vi "Multipoint SMU Read.vi"() -> ()   [LabVIEW 2010]
uses:
  <instrlib>/Keithley 2400/Keithley 24XX.lvlib
panel:
  out "Waveform Chart":sgl[](graph)
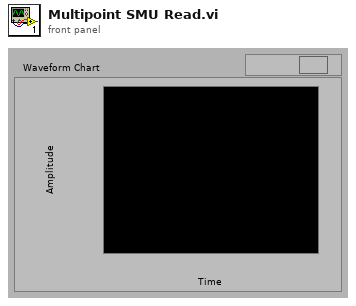
[diagram p1: front panel]
types:
  T1 = enum16{"--Disconnect All--", "Connect PulseGen to CH1", "Connect PulseGen to CH2", "Connect PulseGen to CH3", "Connect PulseGen to CH4", "Connect PulseGen to CH5", "Connect PulseGen to CH6", "Connect PulseGen to CH7", "Connect PulseGen to CH8", "Connect PulseGen to CH9", "Connect PulseGen to CH10", "Connect PulseGen to CH11", "Connect PulseGen to CH12", "Connect PulseGen to CH13", "Connect PulseGen to CH14", "Connect PulseGen to CH15", "Connect PulseGen to CH16", "Connect PulseGen to CH17", "Connect PulseGen to CH18", "Connect PulseGen to CH19", "Connect PulseGen to CH20", "Connect PulseGen to CH21", "Connect PulseGen to CH22", "Connect PulseGen to CH23", "Connect PulseGen to CH24", "Connect PulseGen to CH25", "Set MAG_SW", "Set Dynamic Load", "Set Expansion Trigger", "Trigger Positive Pulse", "Trigger Negative Pulse", "Set MSP Magic Pin", "Set BAT_EN", "Connect MSP_ACLK to CTR", "Connect MSP_MCLK to CTR", "Connect MSP_DIG_TST_OUT to CTR", "Connect STIM_SCK to CTR", "Connect STIM_CLK to CTR", "Connect SMU2 to Magnet", "Magnet Enable", "Cap Short", "Connect Positive Pulse to Pulse Bus", "Connect Negative Pulse to Pulse Bus", "Connect JTAG", "Connect JTAG DVDD Power", "RF Attach", "Connect SMU3 to VBAT", "Connect SMU3 Soft Start", "Connect ARB to Charge Coil", "Connect ARB to Matrix", "Connect CTR to Matrix", "DMM_I Short", "DMM_I 1000 Ohm", "DMM_I 100 Ohm", "DMM_I 10 Ohm", "Connect CH25 to DUT GND"}
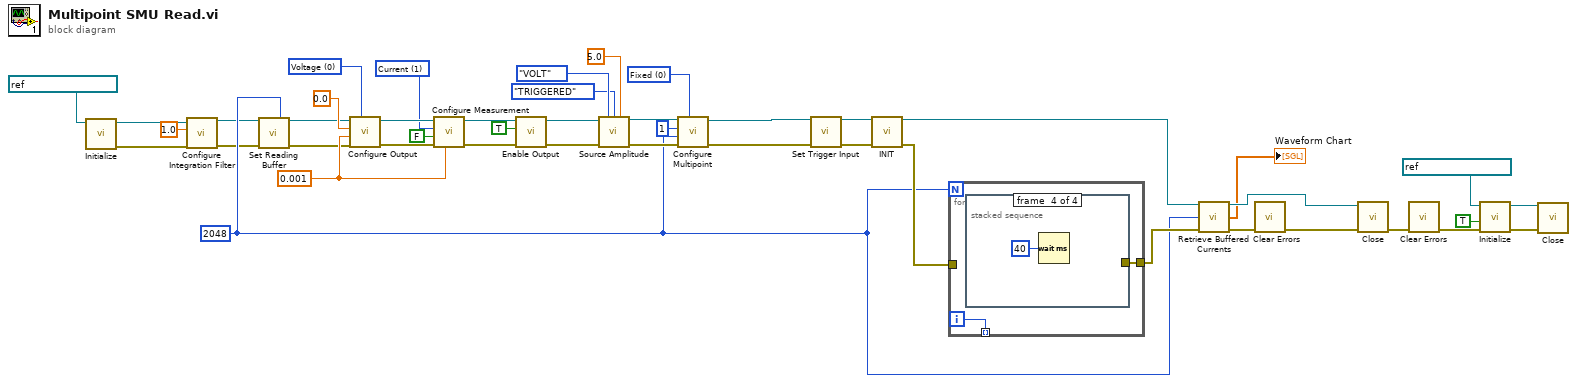
[diagram p0: block diagram]
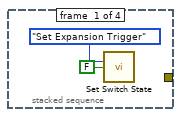
[diagram p2: hidden frame]
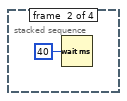
[diagram p3: hidden frame]
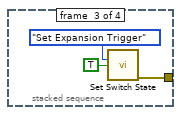
[diagram p4: hidden frame]
diagram:
  w3 = 2048 ("Reading Count")
  w26 = u16 0 items=["Fixed", "Sweep", "List"] ("Output Mode (0: Fixed)")
  w33 = u16 1 items=["Volts", "Current", "Resistance"] ("Function (0: Volts)")
  w34 = u16 0 items=["Voltage", "Current"] ("Source Mode  (0: Voltage)")
  w31 = 0.001 ("Compliance  Level (0.1)")
  n1 = call <instrlib>:"Initialize.vi"("VISA resource name"=refnum<visa-resource-name> "GPIB0::9::INSTR") -> ("error out"=w43:errorcluster, "VISA resource name out"=w45:refnum<visa-resource-name>)  [unwired: 9 in]
  n2 = call <instrlib>:"Configure Integration Filter.vi"("error in (no error)"=w43, "Measurement Speed (1 PLC)"=1.0, "VISA resource name"=w45) -> ("error out"=w1:errorcluster, "VISA resource name out"=w2:refnum<visa-resource-name>)  [unwired: 7 in]
  n3 = call "Set Reading Buffer.vi"("VISA resource name"=w2, "Reading Count"=w3, "error in (no error)"=w1) -> ("VISA resource name out"=w8:refnum<visa-resource-name>, "error out"=w7:errorcluster)  [unwired: 11 in]
  n4 = call <instrlib>:"Configure Output.vi"("Source Mode  (0: Voltage)"=w34, "error in (no error)"=w7, "Compliance  Level (0.1)"=w31, "Output Level (0)"=0.0, "VISA resource name"=w8) -> ("error out"=w41:errorcluster, "VISA resource name out"=w38:refnum<visa-resource-name>)  [unwired: 5 in]
  n5 = call <instrlib>:"Configure Measurement.vi"("Manual Range (1.0)"=w31, "error in (no error)"=w41, "Enable Auto Range (T:Enable)"=FALSE, "Function (0: Volts)"=w33, "VISA resource name"=w38) -> ("error out"=w40:errorcluster, "VISA resource name out"=w37:refnum<visa-resource-name>)  [unwired: 5 in]
  n6 = call <instrlib>:"Enable Output.vi"("error in (no error)"=w40, "Enable Output (T: Enable)"=TRUE, "VISA resource name"=w37) -> ("error out"=w39:errorcluster, "VISA resource name out"=w36:refnum<visa-resource-name>)  [unwired: 7 in]
  n7 = call "Source Amplitude.vi"("VISA resource name"=w36, "Source Function"=enum16{"CURR", "VOLT"}."VOLT", "Mode"=enum16{"IMM", "TRIGGERED"}."TRIGGERED", "Source Level"=5.0, "error in (no error)"=w39) -> ("VISA resource name out"=w25:refnum<visa-resource-name>, "error out"=w24:errorcluster)  [unwired: 9 in]
  n8 = call <instrlib>:"Configure Multipoint.vi"("Output Mode (0: Fixed)"=w26, "error in (no error)"=w24, "Trigger Count (1)"=w3, "Number of Times to Arm (1)"=1, "VISA resource name"=w25) -> ("error out"=w5:errorcluster, "VISA resource name out"=w6:refnum<visa-resource-name>)  [unwired: 5 in]
  n9 = call "Set Trigger Input.vi"("VISA resource name"=w6, "error in (no error)"=w5) -> ("VISA resource name out"=w21:refnum<visa-resource-name>, "error out"=w20:errorcluster)  [unwired: 12 in]
  n10 = call "INIT.vi"("VISA resource name"=w21, "error in (no error)"=w20) -> ("VISA resource name out"=w9:refnum<visa-resource-name>, "error out"=w23:errorcluster)  [unwired: 12 in]
  n11 = for {
    N: w3 -> [_]
    tunnel: [w47] -> w10
    tunnel: w23 -> [_]
    tunnel: [w46] -> _ mode=indexing
    i -> [w46]
    n12 = stacked-sequence {
      tunnel: [_ _ w51 _] -> w47
      frame #0 {
        n13 = call "Set Switch State.vi"("Action"=T1."Set Expansion Trigger", "State"=FALSE) -> ()  [unwired: 13 in, 1 out]
      }
      frame #1 {
        n14 = Wait (ms)(milliseconds to wait=u32 40) -> ()  [unwired: 1 out]
      }
      frame #2 {
        n15 = call "Set Switch State.vi"("Action"=T1."Set Expansion Trigger", "State"=TRUE) -> ("error out"=w51:errorcluster)  [unwired: 13 in]
      }
      frame #3 {
        n16 = Wait (ms)(milliseconds to wait=u32 40) -> ()  [unwired: 1 out]
      }
    }
  }
  n17 = call "Retrieve Buffered Currents.vi"("VISA resource name in"=w9, "Expected Points?"=w3, "error in"=w10) -> ("VISA resource name out"=w12:refnum<visa-resource-name>, "Current Data"=→"Waveform Chart":sgl[], "error out"=w13:errorcluster)  [unwired: 10 in]
  n18 = call <vilib>:"Clear Errors.vi"("error in (no error)"=w13) -> ("error out"=w11:errorcluster)  [unwired: 6 in]
  n19 = call <instrlib>:"Close.vi"("error in (no error)"=w11, "VISA resource name"=w12) -> ("error out"=w17:errorcluster)  [unwired: 9 in]
  n20 = call <vilib>:"Clear Errors.vi"("error in (no error)"=w17) -> ("error out"=w16:errorcluster)  [unwired: 6 in]
  n21 = call <instrlib>:"Initialize.vi"("error in (no error)"=w16, "Reset (True)"=TRUE, "VISA resource name"=refnum<visa-resource-name> "GPIB0::9::INSTR") -> ("error out"=w14:errorcluster, "VISA resource name out"=w15:refnum<visa-resource-name>)  [unwired: 7 in]
  n22 = call <instrlib>:"Close.vi"("error in (no error)"=w14, "VISA resource name"=w15) -> ()  [unwired: 9 in, 1 out]
